vi "Send Stop Nested Actors.vi"(8 "error in (no error)":errorcluster, 9 "Message Priority (Normal)":T1=enum."Normal", 11 "Message Enqueuer":refnum<class "Message Enqueuer.lvclass">) -> (0 "error out":errorcluster, 3 "Message Enqueuer out":refnum<class "Message Enqueuer.lvclass">)   [LabVIEW 2020, in "Nested Actor.lvlib" / "Stop Nested Actors Msg.lvclass"]
uses:
  Stop Nested Actors Msg.lvclass
  Core/ActorFramework/Message Enqueuer/Message Enqueuer.lvclass
  Core/ActorFramework/Message Enqueuer/Message Priority.ctl
  C:/Users/J63553/Projects/_LabVIEW Community/actor-framework/Core/ActorFramework/Message/Message.lvclass
  Core/ActorFramework/Message Enqueuer/Message Enqueuer.lvclass/Message Enqueuer.ctl
  Core/ActorFramework/Message Priority Queue/Priority Enqueue.vi
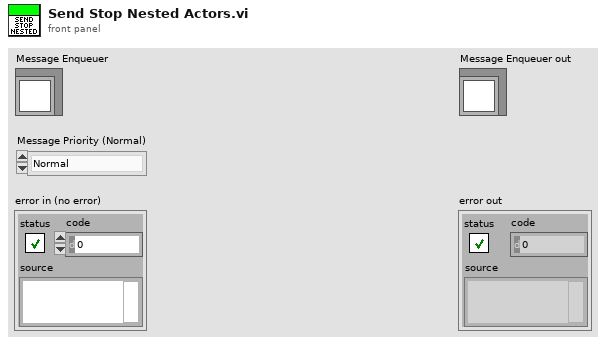
[diagram p1: front panel]
types:
  T1 = typedef "Actor Framework.lvlib/Message Enqueuer.lvclass/Message Priority.ctl" = enum16{"Low", "Normal", "High"}
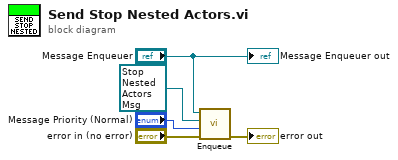
[diagram p0: block diagram]
diagram:
  n1 = call "Enqueue.vi"("error in (no error)"="error in (no error)", "Message Priority (Normal)"="Message Priority (Normal)", "Message"=refnum<class "Stop Nested Actors Msg.lvclass"> refnum ("Report Error Msg in"), "Message Enqueuer in"="Message Enqueuer") -> ("error out"=→"error out":errorcluster)  [unwired: 6 in, 1 out]
  "Message Enqueuer out" <- "Message Enqueuer"
